vi "DMM Instrument UI.vi"() -> ()   [LabVIEW 2025, in "DMM.lvlib" / "DMM Instrument.lvclass"]
doc: "Copyright 2017 National Instruments Corporation\n\nLicensed under the Apache License, Version 2.0 (the \"License\"); you may not use this file except in compliance with the License. You may obtain a copy of the License at http://www.apache.org/licenses/LICENSE-2.0\nUnless required by applicable law or agreed to in writing, software distributed under the License is distributed on an \"AS IS\" BASIS, WITHOUT WARRANTIES OR CONDITIONS OF ANY KIND, either express or implied. See the License for the specific language governing permissions and limitations under the License."
uses:
  DMM Instrument.lvclass
  Users/Public/Documents/Sandia National Labs/TSS Plugin/CEF.lvlibp/Node/NodeRef.ctl
  Users/Public/Documents/Sandia National Labs/TSS Plugin/CEF.lvlibp/Node/CEF_Node.lvclass
  Users/Public/Documents/Sandia National Labs/TSS Plugin/CEF.lvlibp/Node/mainQref.ctl
  Users/Public/Documents/Sandia National Labs/TSS Plugin/CEF.lvlibp/Node/UserEventRef.ctl
  Users/Public/Documents/Sandia National Labs/TSS Plugin/Abstract Engine.lvlibp/Plugin/Abstract/Instrument configuration/Default Instrument.ctl
  DMM configuration/DMM Setting.ctl
  C:/Users/Public/Documents/Sandia National Labs/TSS Plugin/CEF.lvlibp/Node/CEF_Node.lvclass
  DMM Instrument.lvclass/DMM Instrument.ctl
  DMM configuration/DMM configuration.lvclass/DMM configuration.ctl
  DMM configuration/Read DMM Setting.vi
  DMM configuration/Write DMM Setting.vi
  <vilib>/Utility/error.llb/Trim Whitespace One-Sided.vi
  DMM configuration/DMM configuration.lvclass
  C:/Users/Public/Documents/Sandia National Labs/TSS Plugin/Abstract Engine.lvlibp/Plugin/Abstract/Instrument configuration/Instrument configuration.lvclass
  Users/Public/Documents/Sandia National Labs/TSS Plugin/Abstract Engine.lvlibp/Plugin/Abstract/Instrument configuration/Read Instrument Setting.vi
  Users/Public/Documents/Sandia National Labs/TSS Plugin/Abstract Engine.lvlibp/Plugin/Abstract/Instrument configuration/Write Instrument Setting.vi
  Users/Public/Documents/Sandia National Labs/TSS Plugin/Abstract Engine.lvlibp/Plugin/Abstract/Instrument configuration/Instrument configuration.lvclass
panel:
  in  "DMM":cluster{"Default":T1, "Setting":T2}={"Default"={"Type"="Foundation Bus", "Address"="None", "SW Alias"="None", "Description"="* Type = Class", "Enabled"=TRUE}, "Setting"={"Function"="DC Volts", "CurrentSource"="1mA", "Resolution"="5 1/2", "Range"=0.5}} {"Setting"."Range" format="%#_f"}
  in  "user event":T3
  in  "main queue":T4
  in  "node ref":T5
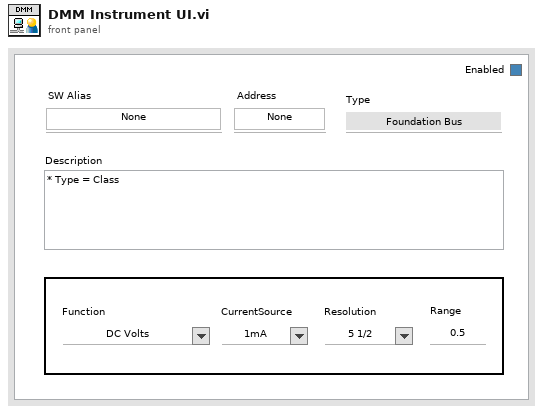
[diagram p1: front panel]
types:
  T1 = typedef "Abstract Engine.lvlibp/Instrument configuration.lvclass/Default Instrument.ctl" = cluster{"Type":string, "Address":string, "SW Alias":string, "Description":string, "Enabled":bool}
  T2 = typedef "DMM.lvlib/DMM configuration.lvclass/DMM Setting.ctl" = cluster{"Function":string, "CurrentSource":string, "Resolution":string, "Range":dbl}
  T3 = typedef "CEF.lvlibp/CEF_Node.lvclass/UserEventRef.ctl" = refnum<user-event>
  T4 = typedef "CEF.lvlibp/CEF_Node.lvclass/mainQref.ctl" = refnum<queue>
  T5 = typedef "CEF.lvlibp/CEF_Node.lvclass/NodeRef.ctl" = refnum<data-value>
  T6 = cluster{"Instrument Setting":T1, "DMM Setting":T2}
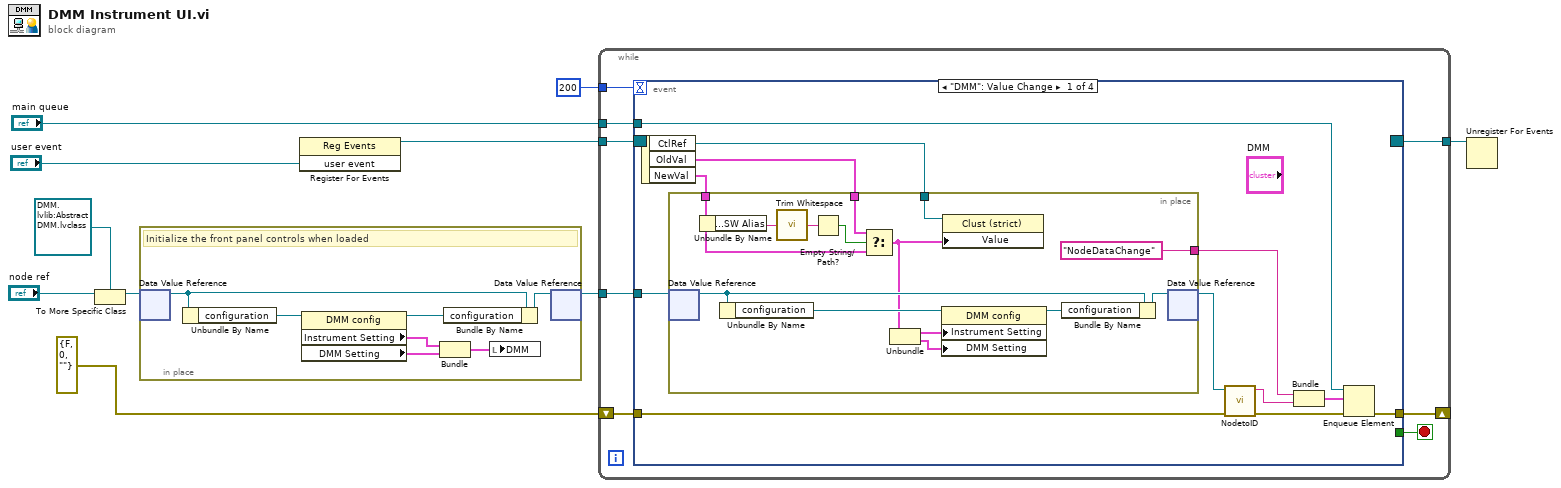
[diagram p0: block diagram]
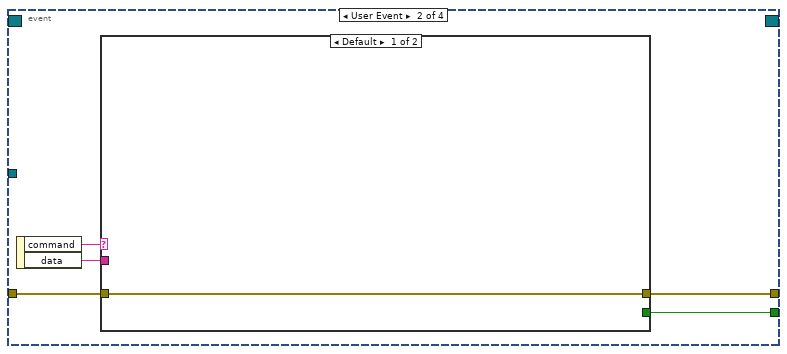
[diagram p2: hidden frame]
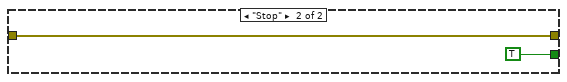
[diagram p3: hidden frame]
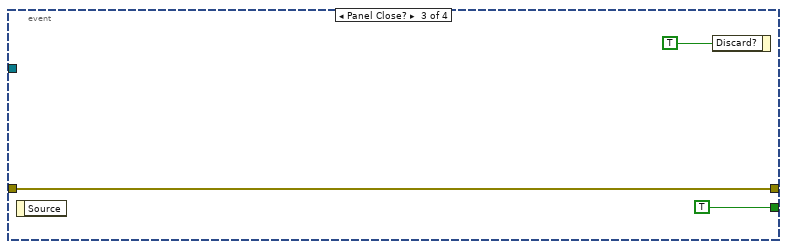
[diagram p4: hidden frame]
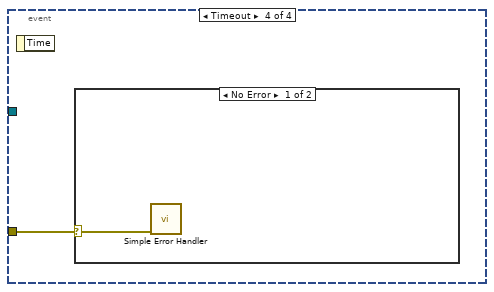
[diagram p5: hidden frame]
diagram:
  n1 = To More Specific Class(target class=refnum<data-value> refnum ("data value reference"), reference="node ref") -> (specific class reference=w6:refnum<data-value>)  [unwired: 1 in, 1 out]
  n2 = in-place {
    # "Initialize the front panel controls when loaded"
    n3 = in-place-dvr #1(w6) -> (w13:refnum<class "DMM Instrument.lvclass">)  [unwired: 1 out]
    n4 = Unbundle By Name(w13) -> ("configuration"=w17:refnum<class "DMM configuration.lvclass">)
    n5 = property class="DMM config"(reference=w17) -> (reference out=w15:refnum<class "DMM configuration.lvclass">, "Instrument Setting"=w12:T1, "DMM Setting"=w11:T2)  [unwired: 1 in, 1 out]
    n6 = Bundle("Instrument Setting"=w12, "DMM Setting"=w11) -> (w14:T6)  [unwired: 1 in]
    n7 = Bundle By Name(cluster=w13, "configuration"=w15) -> (w16:refnum<class "DMM Instrument.lvclass">)
    n8 = local write "DMM"(w14) -> ()
    n9 = in-place-dvr #1(w16) -> (w7:refnum<data-value>)  [unwired: 1 out]
  }
  n10 = register-events("user event") -> (reference out=w4:refnum<event-registration>)  [unwired: 2 in, 1 out]
  n11 = while {
    tunnel: w7 -> [w25]
    tunnel: w4 -> [w23]
    tunnel: [w22] -> w8
    tunnel: "main queue" -> [w20]
    shift-right: [w24] -> _
    shift-left: errorcluster {"status"=FALSE, "code"=0, "source"=""} ("error out") -> [w19]
    tunnel: 200 -> [w18]
    stop <- w21 stop-if-true
    n12 = event shown="[0] \"DMM\": Value Change" {
      selector: w23 -> [_ _ _ _]
      dyn-events: [_ _ _ _] -> w22
      timeout: w18 -> [_ _ _ _]
      tunnel: [w37 w52 w60 _] -> w24
      tunnel: w25 -> [w34 _ _ _]
      tunnel: [_ w55 TRUE _] -> w21
      tunnel: w20 -> [w35 _ _ _]
      tunnel: w19 -> [w29 w53 w60 w63]
      event "DMM": Value Change {
        n13 = event-data() -> ("CtlRef"=w31:refnum<vi>, "OldVal"=w32:cluster{"Default":T1, "Setting":T2}, "NewVal"=w30:cluster{"Default":T1, "Setting":T2})  [unwired: 1 in]
        n14 = in-place {
          in-place-border: w32 -> [w48]
          in-place-border: w31 -> [w47]
          in-place-border: w30 -> [w41]
          in-place-border: ["NodeDataChange" ("Message Name")] -> w27
          n15 = in-place-dvr #2(w34) -> (w51:refnum<class "DMM Instrument.lvclass">)  [unwired: 1 out]
          n16 = Unbundle By Name(w41) -> ("Default.SW Alias"=w40:string)
          n17 = Unbundle By Name(w51) -> ("configuration"=w46:refnum<class "DMM configuration.lvclass">)
          n18 = call <vilib>:"Trim Whitespace.vi"("string"=w40) -> ("trimmed string"=w43:string)  [unwired: 1 in]
          n19 = Empty String/Path?(string/path=w43) -> (empty?=w42:bool)
          n20 = Select(t=w48, s=w42, f=w41) -> (s? t:f=w45:cluster{"Default":T1, "Setting":T2})
          n21 = Unbundle(w45) -> ("Default"=w44:T1, "Setting"=w39:T2)
          n22 = property class="DMM config"(reference=w46, "Instrument Setting"=w44, "DMM Setting"=w39) -> (reference out=w50:refnum<class "DMM configuration.lvclass">)  [unwired: 1 in, 1 out]
          n23 = property class="Clust (strict)"(reference=w47, "Value"=w45) -> ()  [unwired: 1 in, 2 out]
          n24 = Bundle By Name(cluster=w51, "configuration"=w50) -> (w49:refnum<class "DMM Instrument.lvclass">)
          n25 = in-place-dvr #2(w49) -> (w33:refnum<data-value>)  [unwired: 1 out]
        }
        n26 = call "NodetoID.vi"("error in"=w29, "node ref"=w33) -> ("error out"=w36:errorcluster, "ID"=w28:string)  [unwired: 8 in]
        n27 = Bundle("Message Name"=w27, "ID"=w28) -> (w26:cluster{"Message Name":string, "ID":string})  [unwired: 1 in]
        n28 = Enqueue Element(queue=w35, element=w26, error in (no error)=w36) -> (error out=w37:errorcluster)  [unwired: 1 in, 2 out]
      }
      event User Event {
        n29 = event-data() -> ("command"=w54:string, "data"=w56:string)  [unwired: 1 in]
        n30 = case shown="Default" w54 {
          tunnel: w56 -> [_ _]
          tunnel: [_ TRUE] -> w55
          tunnel: w53 -> [w57 w58]
          tunnel: [w57 w58] -> w52
          frame Default {
          }
          frame "Stop" {
          }
        }
      }
      event Panel Close? {
        n31 = event-data() -> ()  [unwired: 1 in, 1 out]
        n32 = event-data("Discard?"=TRUE) -> ()  [unwired: 1 in, 1 out]
      }
      event Timeout {
        n33 = event-data() -> ()  [unwired: 1 in, 1 out]
        n34 = case shown="No Error" w63 {
          selector: w63 -> [w64 _]
          frame No Error {
            n35 = call <vilib>:"Simple Error Handler.vi"("error in (no error)"=w64) -> ()  [unwired: 4 in, 5 out]
          }
          frame Error {
          }
        }
      }
    }
  }
  n36 = Unregister For Events(event registration refnum=w8) -> ()  [unwired: 1 in, 1 out]
